vi "TargetMet.vi"(0 "Target x (mm)":dbl, 5 "Target y (mm)":dbl, 7 "Current x (mm)":dbl, 9 "Current y (mm)":dbl, 11 "Dead Zone (mm)":dbl) -> (4 "out":i32)   [LabVIEW 2017, in "controllerLibrary.lvlib"]
doc: "This VI determines if the target has been reached\n\nThe output is 1 if target reahced,\n\notherwise output is zero"
uses:
  controllerLibrary.lvlib
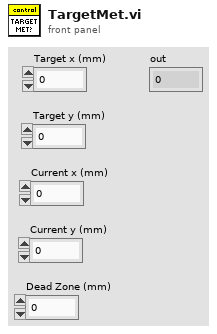
[diagram p1: front panel]
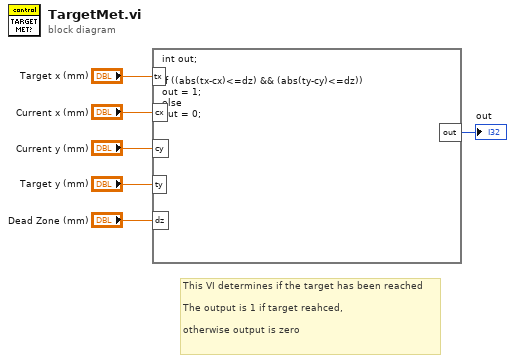
[diagram p0: block diagram]
diagram:
  # "This VI determines if the target has been reached\n\nThe output is 1 if target reahced,\n\notherwise output is zero"
  n1 = formula code="int out;\n\nif ((abs(tx-cx)<=dz) && (abs(ty-cy)<=dz))\nout = 1;\nelse \nout = 0;"("dz"="Dead Zone (mm)", "cx"="Current x (mm)", "cy"="Current y (mm)", "tx"="Target x (mm)", "ty"="Target y (mm)") -> ("out"=→"out":i32)
